vi "Enumerate Ports.vi"(8 "list?":bool=TRUE, 9 "Processor":T1, 11 "Python version":string="3.9") -> (0 "error out":errorcluster, 1 "guess":string, 2 "Short guess":string, 3 "Python":T2, 4 "name":string, 5 "possibilities":string[](array[string]))   [LabVIEW 2022 SP3]
uses:
  PythonCtrl.ctl
  Processors.ctl
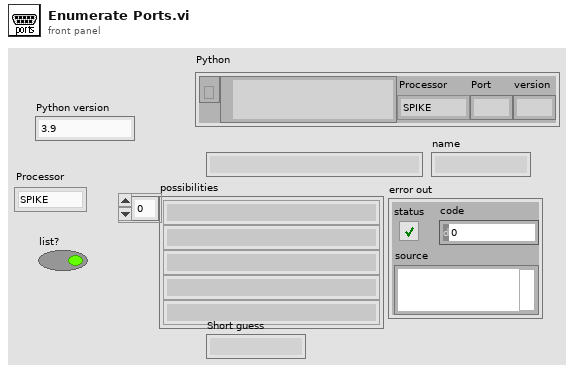
[diagram p1: front panel]
types:
  T1 = typedef "Processors.ctl" = enum16{"SPIKE", "Pi", "Pi_ssh", "OpenMV", "Dunio"}
  T2 = typedef "PythonCtrl.ctl" = cluster{"session":refnum<k35>, "PyPath":path, "Processor":T1, "Port":string, "version":string}
  T3 = cluster{"Refnum out":refnum<k35>, "appended path":path, "Processor":T1, string, "Python version":string}
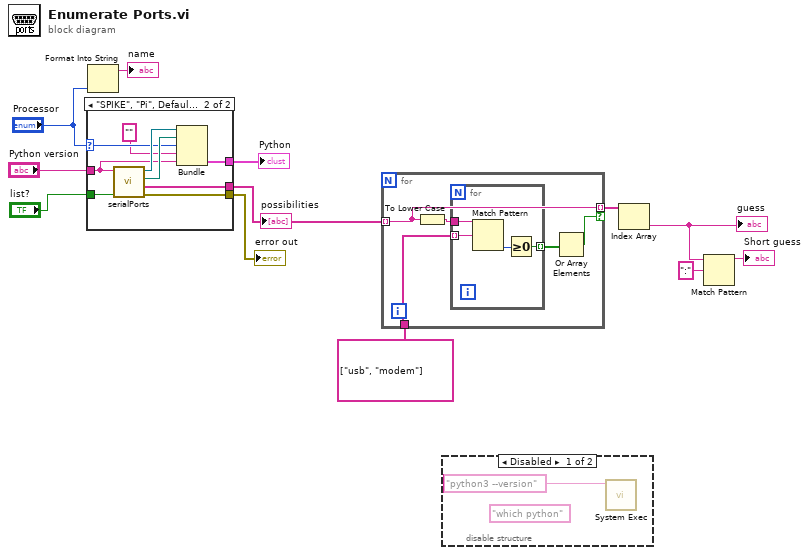
[diagram p0: block diagram]
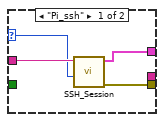
[diagram p2: hidden frame]
diagram:
  n1 = case shown="\"SPIKE\", \"Pi\", Default" "Processor" {
    selector: "Processor" -> [w13 w20]
    tunnel: [_ w25] -> w12
    tunnel: [w14 w24] -> w10
    tunnel: "Python version" -> [w16 w17]
    tunnel: [w15 w21] -> w7
    tunnel: "list?" -> [_ w19]
    frame "Pi_ssh" {
      n2 = call "SSH_Session.vi"("Processor"=w13, "Python version"=w16) -> ("error out"=w14:errorcluster, "Python"=w15:T2)  [unwired: 8 in]
    }
    frame "SPIKE", "Pi", Default {
      n3 = call "serialPorts.vi"("list?"=w19, "Python version"=w17) -> ("error out"=w24:errorcluster, "ports"=w25:string[], "appended path"=w22:path, "Refnum out"=w23:refnum<k35>)  [unwired: 6 in]
      n4 = Bundle("Refnum out"=w23, "appended path"=w22, "Processor"=w20, "", "Python version"=w17) -> (w21:T3)  [unwired: 1 in]
    }
  }
  "possibilities" <- w12
  "error out" <- w10
  "Python" <- w7
  n5 = Format Into String("Processor") -> (resulting string=→"name":string)  [unwired: 3 in, 1 out]
  n6 = for {
    tunnel: w12 -> [w28] mode=indexing
    tunnel: string[] ["usb", "modem"] -> [w30]
    tunnel: [w28] -> w1 mode=indexing if=w27
    n7 = To Lower Case(string=w28) -> (all lower case string=w26:string)
    n8 = for {
      tunnel: w26 -> [w34]
      tunnel: w30 -> [w33] mode=indexing
      tunnel: [w31] -> w29 mode=indexing
      n9 = Match Pattern(string=w34, regular expression=w33) -> (offset past match=w32:i32)  [unwired: 1 in, 3 out]
      n10 = Greater Or Equal To 0?(x=w32) -> (x >= 0?=w31:bool)
    }
    n11 = Or Array Elements(Boolean array=w29) -> (logical OR=w27:bool)
  }
  n12 = disable-structure shown="Disabled" {
    frame Disabled {
      (unwired) "which python" ("command line")
      n13 = call <vilib>:"System Exec.vi"("command line"="python3 --version") -> ()  [unwired: 7 in, 4 out]
    }
    frame Enabled {
    }
  }
  n14 = Index Array(array=w1) -> (element=w4:string)  [unwired: 1 in]
  "guess" <- w4
  n15 = Match Pattern(string=w4, regular expression=":") -> (before substring=→"Short guess":string)  [unwired: 1 in, 3 out]
